vi "Configure Sweep Characteristics.vi"(0 "VISA resource name":refnum<visa-resource-name>, 1 "Sweep Direction (0: Up)":u16(ring) items=["Up", "Down"], 2 "Sweep Type (0: Step)":u16(ring) items=["Step", "List", "Ramp"], 5 "Sweep Mode (0: Off)":u16(ring) items=["Off", "Frequency", "Power", "Frequency and Power"], 7 "Enable Manual Mode (F:Disable)":bool, 9 "Manual Point (1)":i32=1, 11 "error in (no error)":errorcluster, 12 "Manual Frequency (100 kHz)":dbl=100000.0, 13 "Enable Retrace (T:Enable)":bool=TRUE) -> (4 "VISA resource name out":refnum<visa-resource-name>, 15 "error out":errorcluster)   [LabVIEW 2009, in "Agilent PSG MXG Series.lvlib"]
doc: "Configures the sweep type, sweep direction, sweep mode and retrace state of the sweep functions."
uses:
  Agilent PSG MXG Series.lvlib
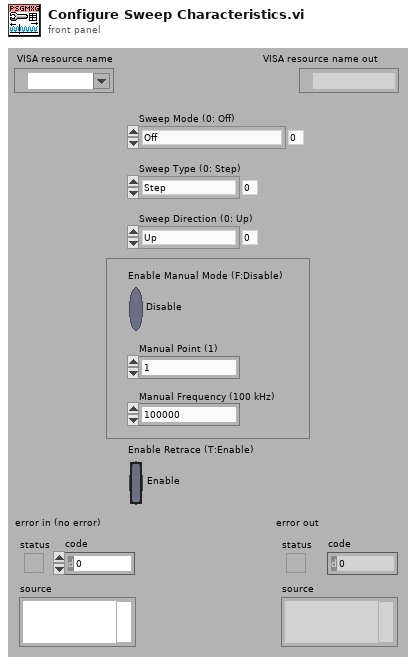
[diagram p1: front panel]
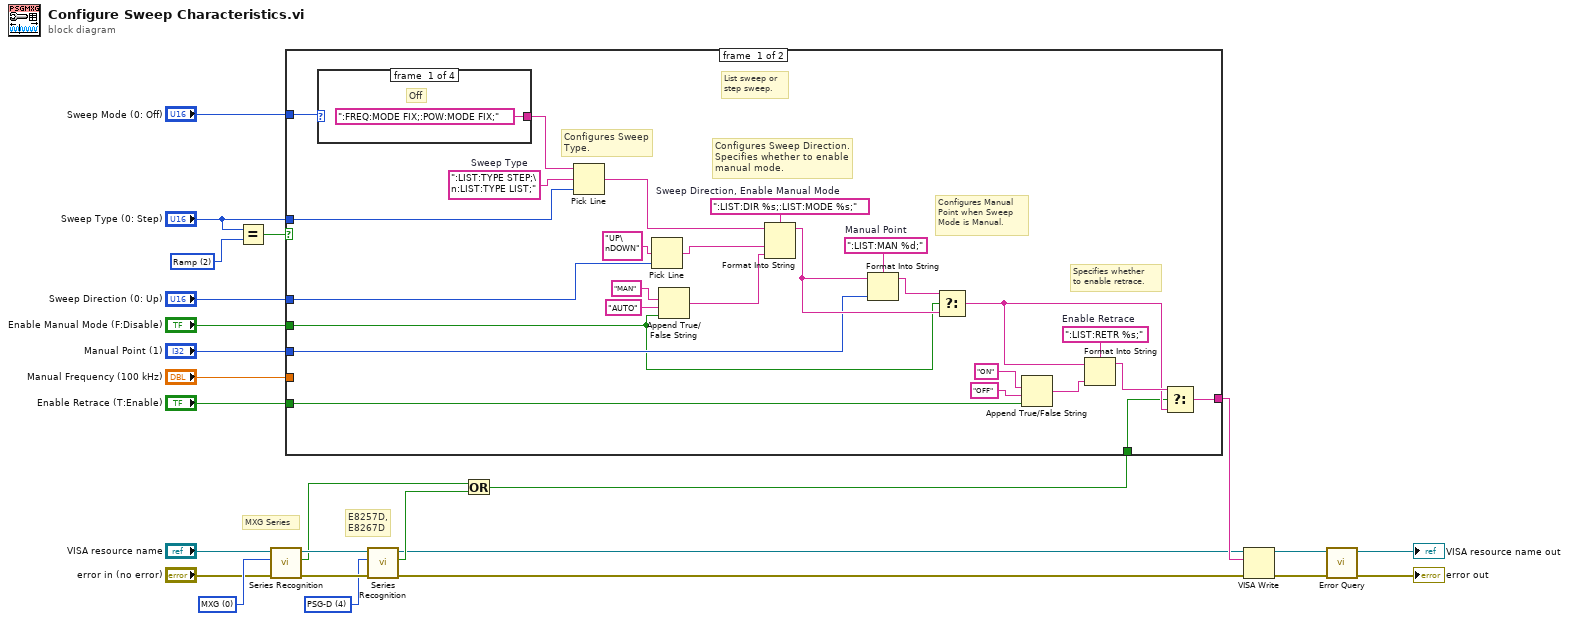
[diagram p0: block diagram]
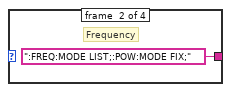
[diagram p2: hidden frame]
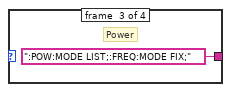
[diagram p3: hidden frame]
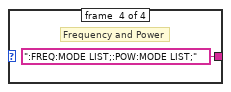
[diagram p4: hidden frame]
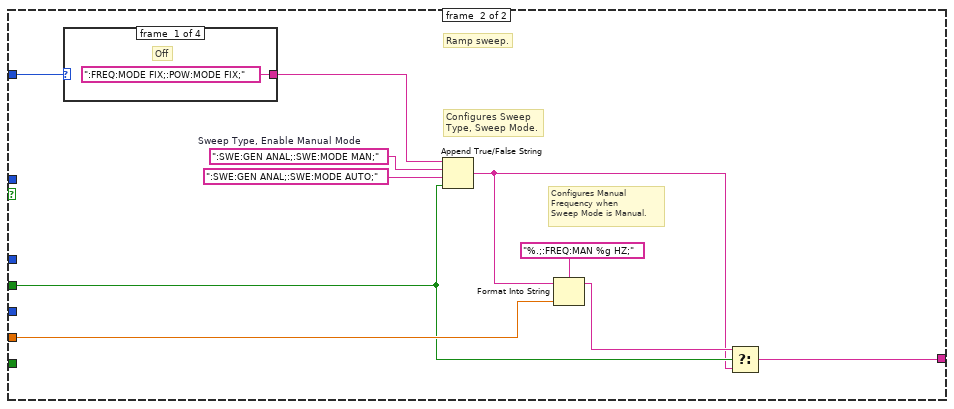
[diagram p5: hidden frame]
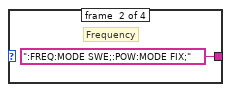
[diagram p6: hidden frame]
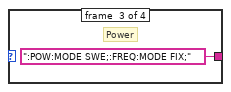
[diagram p7: hidden frame]
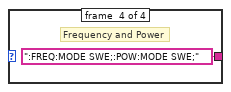
[diagram p8: hidden frame]
diagram:
  w6 = u16 4 items=["MXG", "PSG", "PSG-A", "PSG-C", "PSG-D"] ("Series Type (0: MXG)")
  w7 = u16 0 items=["MXG", "PSG", "PSG-A", "PSG-C", "PSG-D"] ("Series Type (0: MXG)")
  w25 = 2 items=["Step", "List", "Ramp"] ("Sweep Type (0: Step)")
  # "E8257D,\nE8267D"
  # "MXG Series"
  n1 = Equal?(x="Sweep Type (0: Step)", y=w25) -> (x = y?=w24:bool)
  n2 = call "Series Recognition.vi"("error in (no error)"="error in (no error)", "Series Type (0: MXG)"=w7, "VISA resource name"="VISA resource name") -> ("error out"=w13:errorcluster, "Is Series Correct"=w12:bool, "VISA resource name out"=w14:refnum<visa-resource-name>)  [unwired: 1 in, 5 out]
  n3 = call "Series Recognition.vi"("error in (no error)"=w13, "Series Type (0: MXG)"=w6, "VISA resource name"=w14) -> ("error out"=w9:errorcluster, "Is Series Correct"=w11:bool, "VISA resource name out"=w10:refnum<visa-resource-name>)  [unwired: 1 in, 5 out]
  n4 = Or(x=w12, y=w11) -> (x .or. y?=w8:bool)
  n5 = case shown="False" w24 {
    tunnel: "Sweep Type (0: Step)" -> [w50 _]
    tunnel: "Sweep Direction (0: Up)" -> [w46 _]
    tunnel: "Enable Manual Mode (F:Disable)" -> [w27 w57]
    tunnel: "Manual Point (1)" -> [w34 _]
    tunnel: "Manual Frequency (100 kHz)" -> [_ w64]
    tunnel: [w38 w62] -> w18
    tunnel: "Enable Retrace (T:Enable)" -> [w42 _]
    tunnel: "Sweep Mode (0: Off)" -> [w32 w61]
    tunnel: w8 -> [w30 _]
    frame #0 {
      w37 = ":LIST:MAN %d;"  # Manual Point
      w44 = ":LIST:RETR %s;"  # Enable Retrace
      w48 = ":LIST:DIR %s;:LIST:MODE %s;"  # Sweep Direction, Enable Manual Mode
      w51 = ":LIST:TYPE STEP;\n:LIST:TYPE LIST;"  # Sweep Type
      # "Specifies whether\nto enable retrace."
      # "Configures Manual\nPoint when Sweep\nMode is Manual."
      # "Configures Sweep Direction.\nSpecifies whether to enable\nmanual mode."
      # "Configures Sweep\nType."
      # "List sweep or\nstep sweep."
      n6 = case shown="0, Default" w32 {
        tunnel: [":FREQ:MODE FIX;:POW:MODE FIX;" ":FREQ:MODE LIST;:POW:MODE FIX;" ":POW:MODE LIST;:FREQ:MODE FIX;" ":FREQ:MODE LIST;:POW:MODE LIST;"] -> w31
        frame #0 {
          # "Off"
        }
        frame #1 {
          # "Frequency"
        }
        frame #2 {
          # "Power"
        }
        frame #3 {
          # "Frequency and Power"
        }
      }
      n7 = Pick Line(string ("")=w31, multi-line string=w51, line index=w50) -> (output string=w49:string)
      n8 = Pick Line(multi-line string="UP\nDOWN", line index=w46) -> (output string=w45:string)  [unwired: 1 out]
      n9 = Append True/False String(1:w27, 2:"AUTO" ("false string"), 3:"MAN" ("true string")) -> (0:w26:string)  [unwired: 1 out]
      n10 = Format Into String(format string=w48, initial string=w49, w45, w26) -> (resulting string=w35:string)  [unwired: 1 in, 1 out]
      n11 = Format Into String(format string=w37, initial string=w35, w34) -> (resulting string=w36:string)  [unwired: 1 in, 1 out]
      n12 = Select(t=w36, s=w27, f=w35) -> (s? t:f=w33:string)
      n13 = Append True/False String(1:w42, 2:"OFF" ("false string"), 3:"ON" ("true string")) -> (0:w43:string)  [unwired: 1 out]
      n14 = Format Into String(format string=w44, initial string=w33, w43) -> (resulting string=w39:string)  [unwired: 1 in, 1 out]
      n15 = Select(t=w39, s=w30, f=w33) -> (s? t:f=w38:string)
    }
    frame #1 {
      w60 = ":SWE:GEN ANAL;:SWE:MODE MAN;"  # Sweep Type, Enable Manual Mode
      # "Configures Manual\nFrequency when\nSweep Mode is Manual."
      # "Configures Sweep\nType, Sweep Mode."
      # "Ramp sweep."
      n16 = case shown="1" w61 {
        tunnel: [":FREQ:MODE FIX;:POW:MODE FIX;" ":FREQ:MODE SWE;:POW:MODE FIX;" ":POW:MODE SWE;:FREQ:MODE FIX;" ":FREQ:MODE SWE;:POW:MODE SWE;"] -> w58
        frame #0 {
          # "Off"
        }
        frame #1 {
          # "Frequency"
        }
        frame #2 {
          # "Power"
        }
        frame #3 {
          # "Frequency and Power"
        }
      }
      n17 = Append True/False String(1:w57, 2:":SWE:GEN ANAL;:SWE:MODE AUTO;" ("false string"), 3:w60, 4:w58) -> (0:w56:string)
      n18 = Format Into String(format string="%.;:FREQ:MAN %g HZ;", initial string=w56, w64) -> (resulting string=w63:string)  [unwired: 1 in, 1 out]
      n19 = Select(t=w63, s=w57, f=w56) -> (s? t:f=w62:string)
    }
  }
  n20 = VISA Write(VISA resource name=w10, write buffer=w18, error in (no error)=w9) -> (VISA resource name out=w17:refnum<visa-resource-name>, error out=w16:errorcluster)  [unwired: 1 out]
  n21 = call "Error Query.vi"("error in (no error)"=w16, "VISA resource name"=w17) -> ("error out"=→"error out":errorcluster, "VISA resource name out"=→"VISA resource name out":refnum<visa-resource-name>)  [unwired: 8 out]
